vi "Deadzone.vi"(10 "Input":dbl, 11 "Deadzone":dbl) -> (3 "Corected":dbl)   [LabVIEW 2014]
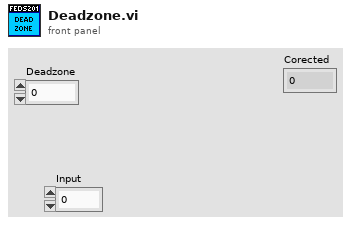
[diagram p1: front panel]
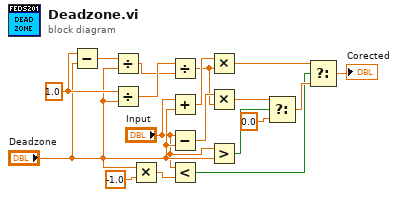
[diagram p0: block diagram]
diagram:
  w7 = 1.0 ("x")
  n1 = Subtract(x=w7, y="Deadzone") -> (x-y=w8:dbl)
  n2 = Divide(x=w8, y="Deadzone") -> (x/y=w1:dbl)
  n3 = Divide(x=w7, y="Deadzone") -> (x/y=w2:dbl)
  n4 = Multiply(x="Deadzone", y=-1.0) -> (x*y=w17:dbl)
  n5 = Divide(x=w2, y=w1) -> (x/y=w6:dbl)
  n6 = Add(x="Input", y="Deadzone") -> (x+y=w10:dbl)
  n7 = Subtract(x="Input", y="Deadzone") -> (x-y=w12:dbl)
  n8 = Less?(x="Input", y=w17) -> (x < y?=w14:bool)
  n9 = Multiply(x=w10, y=w6) -> (x*y=w9:dbl)
  n10 = Multiply(x=w12, y=w6) -> (x*y=w11:dbl)
  n11 = Greater?(x="Input", y="Deadzone") -> (0:w13:bool)
  n12 = Select(t=w11, s=w13, f=0.0) -> (s? t:f=w15:dbl)
  n13 = Select(t=w9, s=w14, f=w15) -> (s? t:f=→"Corected":dbl)
